vi "VoltsToResistance.vi"(2 "Voltage":dbl format="%#_13g", 3 "Bridge settings":T1) -> (1 "Resistance / Ohms":dbl=25.0 format="%0.2f")   [LabVIEW 2014]
uses:
  controls/BridgeSettings.ctl
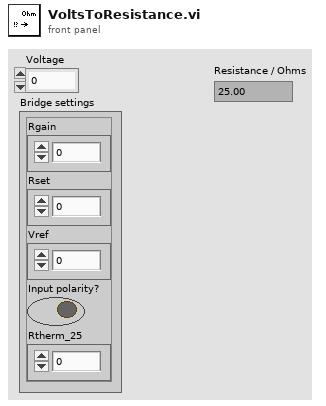
[diagram p1: front panel]
types:
  T1 = typedef "BridgeSettings.ctl" = cluster{"Rgain":dbl, "Rset":dbl, "Vref":dbl, "Input polarity?":bool, "Rtherm_25":dbl}
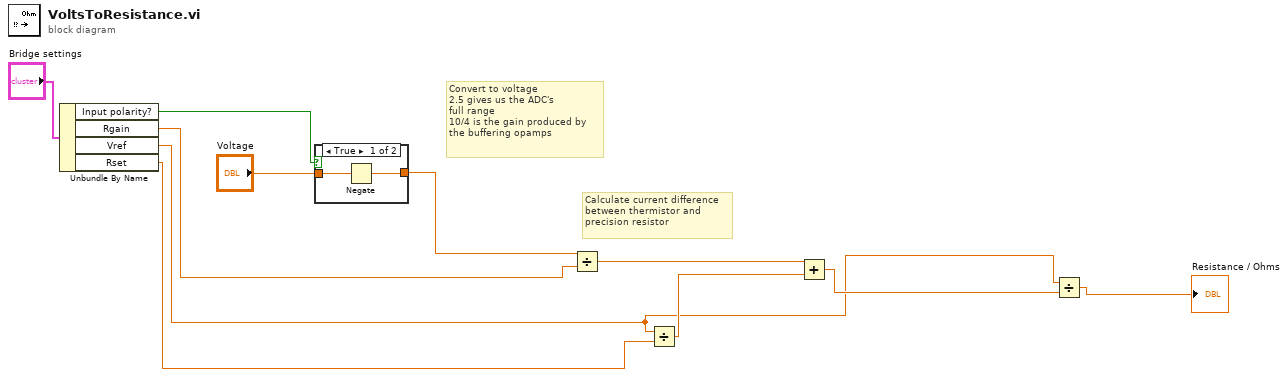
[diagram p0: block diagram]
diagram:
  # "Calculate current difference\nbetween thermistor and\nprecision resistor"
  # "Convert to voltage\n2.5 gives us the ADC's \nfull range\n10/4 is the gain produced by \nthe buffering opamps"
  n1 = Unbundle By Name("Bridge settings") -> ("Input polarity?"=w6:bool, "Rgain"=w5:dbl, "Vref"=w4:dbl, "Rset"=w3:dbl)
  n2 = case shown="True" w6 {
    tunnel: [w12 w14] -> w1
    tunnel: "Voltage" -> [w13 w14]
    frame True {
      n3 = Negate(x=w13) -> (-x=w12:dbl)
    }
    frame False {
    }
  }
  n4 = Divide(x=w1, y=w5) -> (x/y=w11:dbl)
  n5 = Divide(x=w4, y=w3) -> (x/y=w10:dbl)
  n6 = Add(x=w11, y=w10) -> (x+y=w8:dbl)
  n7 = Divide(x=w4, y=w8) -> (x/y=→"Resistance / Ohms":dbl)
